vi "Do.vi"(8 "error in":errorcluster, 10 "Actor in":refnum<class "Actor.lvclass">, 11 "Change Laser Input":refnum<class "Change Laser Input.lvclass">) -> (0 "error out":errorcluster, 2 "Actor out":refnum<class "Actor.lvclass">)   [LabVIEW 2014, in "Change Laser Input.lvclass"]
doc: "(<B>Filename</B>: Actor Framework.lvlib:Message.lvclass:Do.vi)\n\nDefines what a message does when it is received by an actor. Generally, a message instructs an actor to invoke one of its methods. By default, this method does nothing. A child class must override it to define behavior. Create a child class by using the Actor Framework Message Maker dialog box."
uses:
  Change Laser Input.lvclass
  <vilib>/ActorFramework/Actor/Actor.lvclass
  Instr Actor.lvclass
  Instr Actor.lvclass/Instr Actor.ctl
  PAS/Instrument/ePAS.lvclass
  Accessors/Read Instr.vi
  reusable/Instrument/Instrument.lvclass
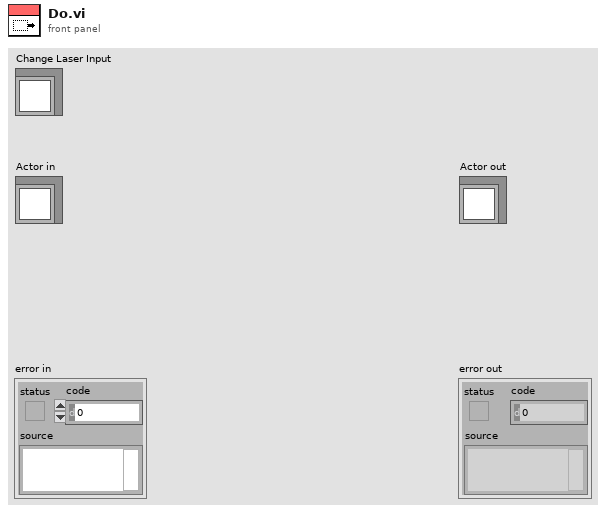
[diagram p1: front panel]
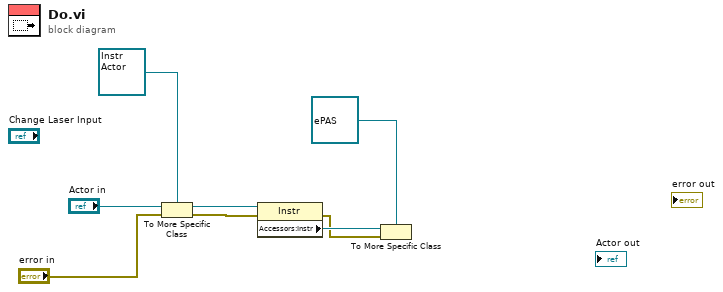
[diagram p0: block diagram]
diagram:
  n1 = To More Specific Class(target class=refnum<class "Instr Actor.lvclass"> refnum ("Instrument Lib:Instr"), reference="Actor in", error in="error in") -> (specific class reference=w6:refnum<class "Instr Actor.lvclass">, error out=w5:errorcluster)
  n2 = property class="Instr"(reference=w6, error in=w5) -> (error out=w2:errorcluster, "Accessors:Instr"=w4:refnum<class "Instrument.lvclass">)  [unwired: 1 out]
  n3 = To More Specific Class(target class=refnum<class "ePAS.lvclass"> refnum ("ePAS"), reference=w4, error in=w2) -> ()  [unwired: 2 out]
